vi "Gyro.vi"() -> (3 "Data Out":u8[](array[numeric]))   [LabVIEW 2018]
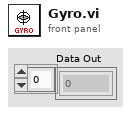
[diagram p1: front panel]
types:
  T1 = typedef "WPI_I2CDevRef.ctl" = cluster{"DevStatus":errorcluster, "Device Address":u8, "Handle":i32, "I2C Bus":T2}
  T2 = typedef "i2c_bus.ctl" = enum16{"I2C On-Board", "I2C MXP", "Invalid"}
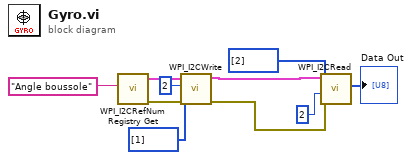
[diagram p0: block diagram]
diagram:
  n1 = call <vilib>:"WPI_I2CRefNum Registry Get.vi"("refnum name"="Angle boussole") -> ("error out"=w5:errorcluster, "I2CDevRef"=w6:T1)  [unwired: 9 in]
  n2 = call <vilib>:"WPI_I2CWrite.vi"("error in (no error)"=w5, "I2CDataToSend"=u8[] [1], "I2CRegister"=u8 2, "I2CDevRef"=w6) -> ("error out"=w4:errorcluster, "I2CDevRef"=w3:T1)  [unwired: 6 in]
  n3 = call <vilib>:"WPI_I2CRead.vi"("error in (no error)"=w4, "I2CBytesToRead"=u8 2, "I2CRegister"=u8[] [2], "I2CDevRef"=w3) -> ("Data Out"=→"Data Out":u8[])  [unwired: 5 in, 2 out]
